vi "FTW-Test-JSON-Fuzz.vi"() -> (0 "Test Result":errorcluster)   [LabVIEW 2014]
uses:
  src/core/error/FTW-ERR-Assert-DeveloperError.vi
  src/core/error/FTW-ERR-ThrowError.vi
  src/core/error/FTW-ERR-CallChain.vi
  src/core/string/FTW-STR-ReplaceWhitespace.vi
  src/core/sync/barrier/FTW-Sync-Synchronizer.xnode
panel:
  out "JSON String (UTF-8)":string
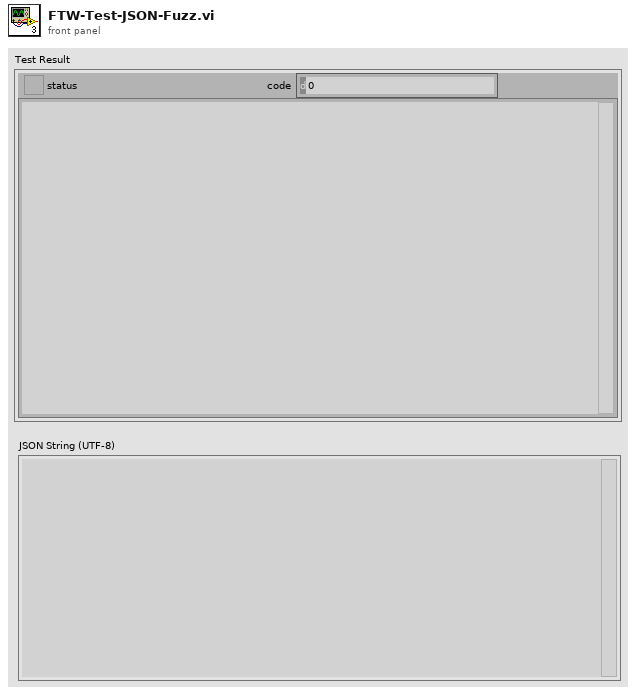
[diagram p1: front panel]
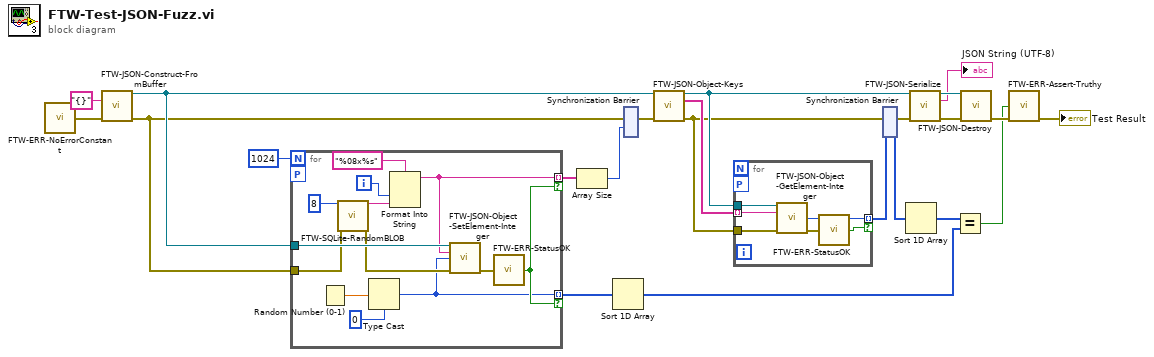
[diagram p0: block diagram]
diagram:
  n1 = call "FTW-ERR-NoErrorConstant.vi"() -> ("no error"=w18:errorcluster)
  n2 = call "FTW-JSON-Construct-FromBuffer.vi"("JSON String (UTF-8)"="{}", "error in"=w18) -> ("JSON Object"=w21:refnum<data-value>, "error out"=w17:errorcluster)  [unwired: 12 in]
  n3 = for {
    N: 1024 -> [_]
    workers-P: _ -> [_]
    tunnel: w17 -> [w34]
    tunnel: w21 -> [w36]
    tunnel: [w25] -> w12 mode=indexing if=w27
    tunnel: [w28] -> w14 mode=indexing if=w27
    i -> [w30]
    n4 = Random Number (0-1)() -> (number: 0 to 1=w26:dbl)
    n5 = call "FTW-SQLite-RandomBLOB.vi"("Number of Bytes"=8, "error in"=w34) -> ("Random BLOB"=w31:string, "error out"=w33:errorcluster)  [unwired: 12 in]
    n6 = Type Cast(type=i64 0, x=w26) -> (*(type *) &x=w25:i64)
    n7 = Format Into String(format string="%08x%s", w30, w31) -> (resulting string=w28:string)  [unwired: 2 in, 1 out]
    n8 = call "FTW-JSON-Object-SetElement-Integer.vi"("JSON Object"=w36, "Key"=w28, "Value"=w25, "error in"=w33) -> ("error out"=w32:errorcluster)  [unwired: 10 in, 1 out]
    n9 = call "FTW-ERR-StatusOK.vi"("error to check"=w32) -> ("Status OK?"=w27:bool)
  }
  n10 = Array Size(array=w14) -> (size(s)=w15:i32)
  n11 = Sort 1D Array(array=w12) -> (sorted array=w10:i64[])
  n12 = xnode "Synchronization Barrier"("Synchronized Signal 1"=w17, "Synchronized Signal 2"=w15) -> ("error out out"=w16:errorcluster)  [unwired: 1 out]
  n13 = call "FTW-JSON-Object-Keys.vi"("JSON Object"=w21, "error in"=w16) -> ("JSON Object out"=w5:refnum<data-value>, "Keys"=w13:string[], "error out"=w4:errorcluster)  [unwired: 11 in]
  n14 = for {
    tunnel: w13 -> [w41] mode=indexing
    tunnel: [w39] -> w1 mode=indexing if=w37
    workers-P: _ -> [_]
    tunnel: w5 -> [w42]
    tunnel: w4 -> [w40]
    n15 = call "FTW-JSON-Object-GetElement-Integer.vi"("JSON Object"=w42, "Key"=w41, "error in"=w40) -> ("Value"=w39:i64, "error out"=w38:errorcluster)  [unwired: 9 in, 2 out]
    n16 = call "FTW-ERR-StatusOK.vi"("error to check"=w38) -> ("Status OK?"=w37:bool)
  }
  n17 = xnode "Synchronization Barrier"("Synchronized Signal 1"=w4, "Synchronized Signal 2"=w1) -> ("error out out"=w3:errorcluster, "out"=w2:i64[])
  n18 = Sort 1D Array(array=w2) -> (sorted array=w11:i64[])
  n19 = call "FTW-JSON-Serialize.vi"("JSON Object"=w5, "error in"=w3) -> ("JSON Object out"=w8:refnum<data-value>, "JSON String (UTF-8)"=→"JSON String (UTF-8)":string, "error out"=w7:errorcluster)  [unwired: 11 in]
  n20 = Equal?(x=w11, y=w10) -> (x = y?=w9:bool)
  n21 = call "FTW-JSON-Destroy.vi"("JSON Object"=w8, "error in"=w7) -> ("error out"=w20:errorcluster)  [unwired: 13 in]
  n22 = call "FTW-ERR-Assert-Truthy.vi"("Expected Truthy"=w9, "error in"=w20) -> ("error out"=→"Test Result":errorcluster)  [unwired: 13 in]
